vi "3-5.vi"() -> ()   [LabVIEW 2017]
panel:
  out "Address":string
  out "Student?":bool
  out "Age":dbl
  out "Name":string
  out "Address 2":string
  out "Name 2":string
  in  "Applicant Cluster":T1
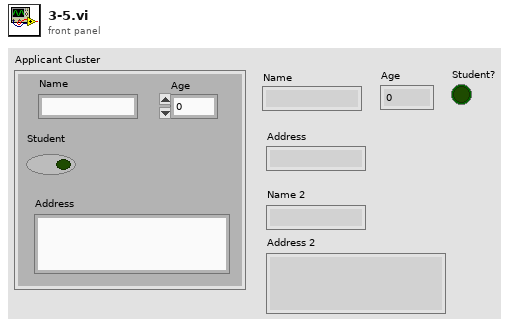
[diagram p1: front panel]
types:
  T1 = cluster{"Name":string, "Age":dbl, "Student":bool, "Address":string}
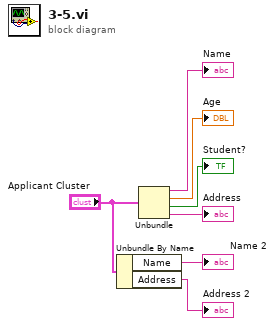
[diagram p0: block diagram]
diagram:
  n1 = Unbundle By Name "Unbundle By Name"("Applicant Cluster") -> ("Name"=→"Name 2":string, "Address"=→"Address 2":string)
  n2 = Unbundle "Unbundle"("Applicant Cluster") -> ("Name"=→"Name":string, "Age"=→"Age":dbl, "Student"=→"Student?":bool, "Address"=→"Address":string)
